vi "TrajectoryBegin.vi"(8 "error in (no error)":errorcluster) -> (0 "error out":errorcluster)   [LabVIEW 2023]
uses:
  TrajectoryGlobals.vi
  <vilib>/Rock Robotics/WPI/ThirdParty/JAS_Junk/TrajLib/Trajectory_Library.lvlib
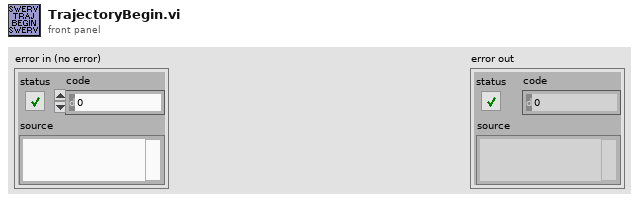
[diagram p1: front panel]
types:
  T1 = typedef "Trajectory_Library.lvlib/TRAJECTORY.ctl" = cluster{"TotalTImeSecs":dbl, "States":T2[]}
  T2 = typedef "Trajectory_Library.lvlib/TRAJ_STATE.ctl" = cluster{"TimeSeconds":dbl, "Velocity":dbl, "Acceleration":dbl, "POSE":T3, "Curvature":dbl}
  T3 = typedef "Trajectory_Library.lvlib/POSE2D.ctl" = cluster{"TRANSLATION":T4, "ROTATION":T5}
  T4 = typedef "Trajectory_Library.lvlib/TRANSLATION2D.ctl" = cluster{"X":dbl, "Y":dbl}
  T5 = typedef "Trajectory_Library.lvlib/ROTATION2D.ctl" = cluster{"VALUE":dbl, "COS":dbl, "SIN":dbl}
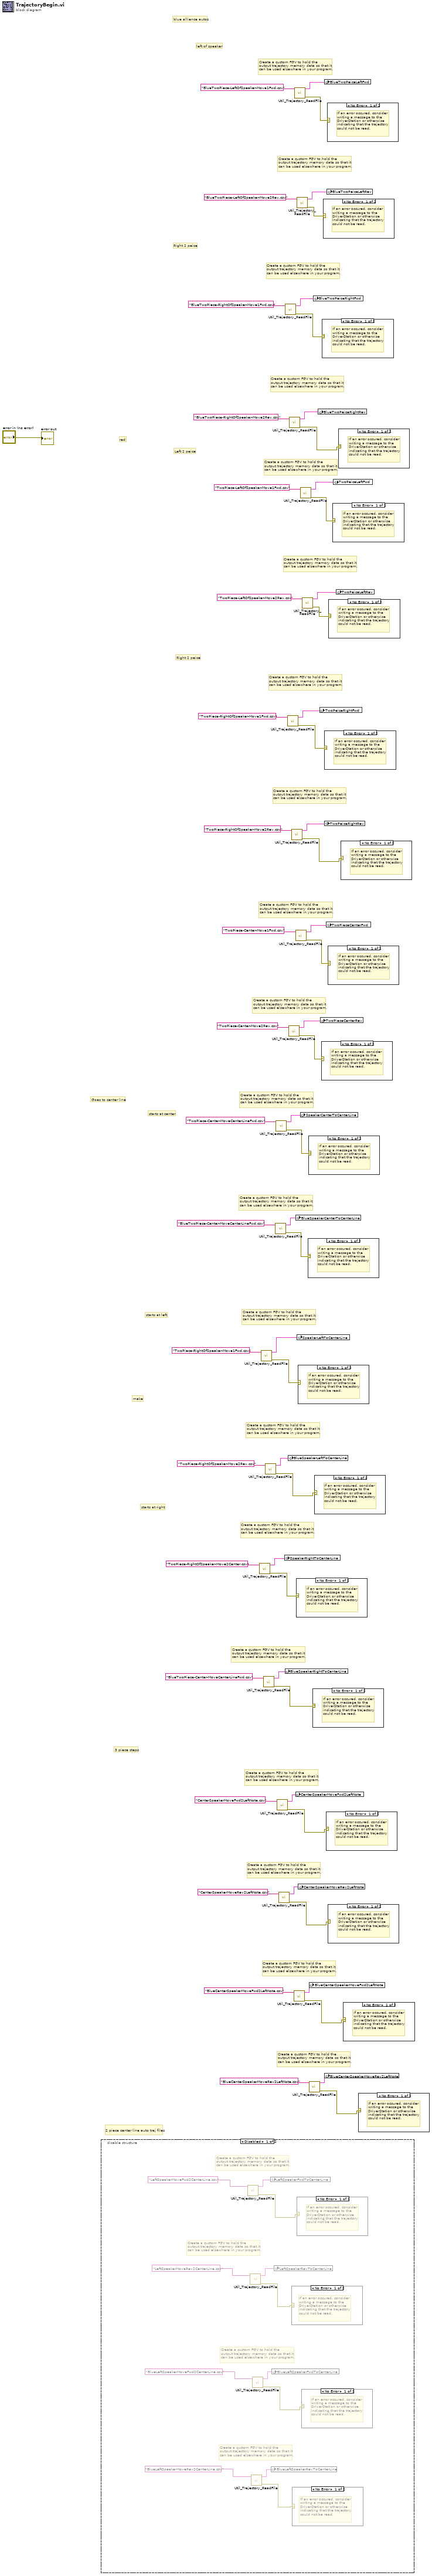
[diagram p0: block diagram]
diagram:
  # "2 piece center line auto traj files"
  # "Create a custom FGV to hold the \noutput trajectory memory data so that it\ncan be used elsewhere in your program."
  # "Create a custom FGV to hold the \noutput trajectory memory data so that it\ncan be used elsewhere in your program."
  # "Create a custom FGV to hold the \noutput trajectory memory data so that it\ncan be used elsewhere in your program."
  # "3 piece steps"
  # "Create a custom FGV to hold the \noutput trajectory memory data so that it\ncan be used elsewhere in your program."
  # "make"
  # "Create a custom FGV to hold the \noutput trajectory memory data so that it\ncan be used elsewhere in your program."
  # "Create a custom FGV to hold the \noutput trajectory memory data so that it\ncan be used elsewhere in your program."
  # "Create a custom FGV to hold the \noutput trajectory memory data so that it\ncan be used elsewhere in your program."
  # "Create a custom FGV to hold the \noutput trajectory memory data so that it\ncan be used elsewhere in your program."
  # "starts at right"
  # "starts at left"
  # "starts at center"
  # "Goes to center line"
  # "Create a custom FGV to hold the \noutput trajectory memory data so that it\ncan be used elsewhere in your program."
  # "Create a custom FGV to hold the \noutput trajectory memory data so that it\ncan be used elsewhere in your program."
  # "Create a custom FGV to hold the \noutput trajectory memory data so that it\ncan be used elsewhere in your program."
  # "Create a custom FGV to hold the \noutput trajectory memory data so that it\ncan be used elsewhere in your program."
  # "red"
  # "Right 2 peice"
  # "Create a custom FGV to hold the \noutput trajectory memory data so that it\ncan be used elsewhere in your program."
  # "Create a custom FGV to hold the \noutput trajectory memory data so that it\ncan be used elsewhere in your program."
  # "Create a custom FGV to hold the \noutput trajectory memory data so that it\ncan be used elsewhere in your program."
  # "Create a custom FGV to hold the \noutput trajectory memory data so that it\ncan be used elsewhere in your program."
  # "left of speaker"
  # "blue allience autos"
  # "Right 2 peice"
  # "Left 2 peice"
  # "Create a custom FGV to hold the \noutput trajectory memory data so that it\ncan be used elsewhere in your program."
  # "Create a custom FGV to hold the \noutput trajectory memory data so that it\ncan be used elsewhere in your program."
  # "Create a custom FGV to hold the \noutput trajectory memory data so that it\ncan be used elsewhere in your program."
  # "Create a custom FGV to hold the \noutput trajectory memory data so that it\ncan be used elsewhere in your program."
  n1 = disable-structure shown="Disabled" {
    frame Disabled {
      # "Create a custom FGV to hold the \noutput trajectory memory data so that it\ncan be used elsewhere in your program."
      # "Create a custom FGV to hold the \noutput trajectory memory data so that it\ncan be used elsewhere in your program."
      # "Create a custom FGV to hold the \noutput trajectory memory data so that it\ncan be used elsewhere in your program."
      # "Create a custom FGV to hold the \noutput trajectory memory data so that it\ncan be used elsewhere in your program."
      n2 = call <vilib>:"Util_Trajectory_ReadFile.vi"("FileName"="LeftSpeakerMoveFwd2CenterLine.csv") -> ("error out"=w71:errorcluster, "outTRAJECTORY"=w72:T1)  [unwired: 8 in, 1 out]
      n3 = call <vilib>:"Util_Trajectory_ReadFile.vi"("FileName"="LeftSpeakerMoveRev2CenterLine.csv") -> ("error out"=w68:errorcluster, "outTRAJECTORY"=w69:T1)  [unwired: 8 in, 1 out]
      n4 = call <vilib>:"Util_Trajectory_ReadFile.vi"("FileName"="BlueLeftSpeakerMoveRev2CenterLine.csv") -> ("error out"=w62:errorcluster, "outTRAJECTORY"=w63:T1)  [unwired: 8 in, 1 out]
      n5 = call <vilib>:"Util_Trajectory_ReadFile.vi"("FileName"="BlueLeftSpeakerMoveFwd2CenterLine.csv") -> ("error out"=w65:errorcluster, "outTRAJECTORY"=w66:T1)  [unwired: 8 in, 1 out]
      n6 = global write "TrajectoryGlobals.vi" "LeftSpeakerFwdToCenterLine"(w72) -> ()
      n7 = global write "TrajectoryGlobals.vi" "BlueLeftSpeakerRevToCenterLine"(w63) -> ()
      n8 = global write "TrajectoryGlobals.vi" "BlueLeftSpeakerFwdToCenterLine"(w66) -> ()
      n9 = global write "TrajectoryGlobals.vi" "LeftSpeakerRevToCenterLine"(w69) -> ()
      n10 = case shown="No Error" w68 {
        frame No Error {
          # "If an error occured, consider\nwriting a message to the\nDriverStation or otherwise\nindicating that the trajectory\ncould not be read."
        }
        frame Error {
        }
      }
      n11 = case shown="No Error" w62 {
        frame No Error {
          # "If an error occured, consider\nwriting a message to the\nDriverStation or otherwise\nindicating that the trajectory\ncould not be read."
        }
        frame Error {
        }
      }
      n12 = case shown="No Error" w71 {
        frame No Error {
          # "If an error occured, consider\nwriting a message to the\nDriverStation or otherwise\nindicating that the trajectory\ncould not be read."
        }
        frame Error {
        }
      }
      n13 = case shown="No Error" w65 {
        frame No Error {
          # "If an error occured, consider\nwriting a message to the\nDriverStation or otherwise\nindicating that the trajectory\ncould not be read."
        }
        frame Error {
        }
      }
    }
    frame Enabled {
    }
  }
  n14 = call <vilib>:"Util_Trajectory_ReadFile.vi"("FileName"="TwoPiece-RightOfSpeaker-Move2Center.csv") -> ("error out"=w22:errorcluster, "outTRAJECTORY"=w23:T1)  [unwired: 8 in, 1 out]
  n15 = call <vilib>:"Util_Trajectory_ReadFile.vi"("FileName"="TwoPiece-RightOfSpeaker-Move1Fwd.csv") -> ("error out"=w16:errorcluster, "outTRAJECTORY"=w17:T1)  [unwired: 8 in, 1 out]
  n16 = call <vilib>:"Util_Trajectory_ReadFile.vi"("FileName"="BlueTwoPiece-Center-MoveCenterLineFwd.csv") -> ("error out"=w19:errorcluster, "outTRAJECTORY"=w20:T1)  [unwired: 8 in, 1 out]
  n17 = call <vilib>:"Util_Trajectory_ReadFile.vi"("FileName"="TwoPiece-RightOfSpeaker-Move2Rev.csv") -> ("error out"=w13:errorcluster, "outTRAJECTORY"=w14:T1)  [unwired: 8 in, 1 out]
  n18 = call <vilib>:"Util_Trajectory_ReadFile.vi"("FileName"="BlueTwoPiece-Center-MoveCenterLineFwd.csv") -> ("error out"=w27:errorcluster, "outTRAJECTORY"=w25:T1)  [unwired: 8 in, 1 out]
  n19 = call <vilib>:"Util_Trajectory_ReadFile.vi"("FileName"="TwoPiece-Center-MoveCenterLineFwd.csv") -> ("error out"=w30:errorcluster, "outTRAJECTORY"=w28:T1)  [unwired: 8 in, 1 out]
  n20 = call <vilib>:"Util_Trajectory_ReadFile.vi"("FileName"="CenterSpeakerMoveFwd2LeftNote.csv") -> ("error out"=w10:errorcluster, "outTRAJECTORY"=w11:T1)  [unwired: 8 in, 1 out]
  n21 = call <vilib>:"Util_Trajectory_ReadFile.vi"("FileName"="CenterSpeakerMoveRev2LeftNote.csv") -> ("error out"=w7:errorcluster, "outTRAJECTORY"=w8:T1)  [unwired: 8 in, 1 out]
  n22 = global write "TrajectoryGlobals.vi" "SpeakerRightToCenterLine"(w23) -> ()
  n23 = global write "TrajectoryGlobals.vi" "BlueSpeakerRightToCenterLine"(w20) -> ()
  n24 = call <vilib>:"Util_Trajectory_ReadFile.vi"("FileName"="BlueTwoPiece-RightOfSpeaker-Move1Fwd.csv") -> ("error out"=w40:errorcluster, "outTRAJECTORY"=w41:T1)  [unwired: 8 in, 1 out]
  n25 = call <vilib>:"Util_Trajectory_ReadFile.vi"("FileName"="TwoPiece-RightOfSpeaker-Move1Fwd.csv") -> ("error out"=w52:errorcluster, "outTRAJECTORY"=w53:T1)  [unwired: 8 in, 1 out]
  n26 = global write "TrajectoryGlobals.vi" "BlueSpeakerLeftToCenterLine"(w14) -> ()
  n27 = call <vilib>:"Util_Trajectory_ReadFile.vi"("FileName"="TwoPiece-Center-Move2Rev.csv") -> ("error out"=w33:errorcluster, "outTRAJECTORY"=w31:T1)  [unwired: 8 in, 1 out]
  n28 = call <vilib>:"Util_Trajectory_ReadFile.vi"("FileName"="BlueTwoPiece-RightOfSpeaker-Move2Rev.csv") -> ("error out"=w37:errorcluster, "outTRAJECTORY"=w38:T1)  [unwired: 8 in, 1 out]
  n29 = call <vilib>:"Util_Trajectory_ReadFile.vi"("FileName"="TwoPiece-RightOfSpeaker-Move2Rev.csv") -> ("error out"=w49:errorcluster, "outTRAJECTORY"=w50:T1)  [unwired: 8 in, 1 out]
  n30 = call <vilib>:"Util_Trajectory_ReadFile.vi"("FileName"="BlueCenterSpeakerMoveFwd2LeftNote.csv") -> ("error out"=w4:errorcluster, "outTRAJECTORY"=w5:T1)  [unwired: 8 in, 1 out]
  n31 = call <vilib>:"Util_Trajectory_ReadFile.vi"("FileName"="BlueTwoPiece-LeftOfSpeaker-Move1Fwd.csv") -> ("error out"=w48:errorcluster, "outTRAJECTORY"=w46:T1)  [unwired: 8 in, 1 out]
  n32 = call <vilib>:"Util_Trajectory_ReadFile.vi"("FileName"="TwoPiece-Center-Move1Fwd.csv") -> ("error out"=w36:errorcluster, "outTRAJECTORY"=w34:T1)  [unwired: 8 in, 1 out]
  n33 = global write "TrajectoryGlobals.vi" "CenterSpeakerMoveFwd2LeftNote"(w11) -> ()
  n34 = global write "TrajectoryGlobals.vi" "BlueSpeakerCenterToCenterLine"(w25) -> ()
  n35 = case shown="No Error" w22 {
    frame No Error {
      # "If an error occured, consider\nwriting a message to the\nDriverStation or otherwise\nindicating that the trajectory\ncould not be read."
    }
    frame Error {
    }
  }
  n36 = call <vilib>:"Util_Trajectory_ReadFile.vi"("FileName"="BlueTwoPiece-LeftOfSpeaker-Move2Rev.csv") -> ("error out"=w43:errorcluster, "outTRAJECTORY"=w44:T1)  [unwired: 8 in, 1 out]
  n37 = global write "TrajectoryGlobals.vi" "SpeakerLeftToCenterLine"(w17) -> ()
  n38 = case shown="No Error" w16 {
    frame No Error {
      # "If an error occured, consider\nwriting a message to the\nDriverStation or otherwise\nindicating that the trajectory\ncould not be read."
    }
    frame Error {
    }
  }
  n39 = global write "TrajectoryGlobals.vi" "CenterSpeakerMoveRev2LeftNote"(w8) -> ()
  n40 = call <vilib>:"Util_Trajectory_ReadFile.vi"("FileName"="TwoPiece-LeftOfSpeaker-Move1Fwd.csv") -> ("error out"=w60:errorcluster, "outTRAJECTORY"=w58:T1)  [unwired: 8 in, 1 out]
  n41 = global write "TrajectoryGlobals.vi" "SpeakerCenterToCenterLine"(w28) -> ()
  n42 = call <vilib>:"Util_Trajectory_ReadFile.vi"("FileName"="TwoPiece-LeftOfSpeaker-Move2Rev.csv") -> ("error out"=w55:errorcluster, "outTRAJECTORY"=w56:T1)  [unwired: 8 in, 1 out]
  n43 = case shown="No Error" w27 {
    frame No Error {
      # "If an error occured, consider\nwriting a message to the\nDriverStation or otherwise\nindicating that the trajectory\ncould not be read."
    }
    frame Error {
    }
  }
  n44 = case shown="No Error" w30 {
    frame No Error {
      # "If an error occured, consider\nwriting a message to the\nDriverStation or otherwise\nindicating that the trajectory\ncould not be read."
    }
    frame Error {
    }
  }
  n45 = global write "TrajectoryGlobals.vi" "BlueCenterSpeakerMoveFwd2LeftNote"(w5) -> ()
  n46 = call <vilib>:"Util_Trajectory_ReadFile.vi"("FileName"="BlueCenterSpeakerMoveRev2LeftNote.csv") -> ("error out"=w1:errorcluster, "outTRAJECTORY"=w2:T1)  [unwired: 8 in, 1 out]
  n47 = case shown="No Error" w19 {
    frame No Error {
      # "If an error occured, consider\nwriting a message to the\nDriverStation or otherwise\nindicating that the trajectory\ncould not be read."
    }
    frame Error {
    }
  }
  n48 = global write "TrajectoryGlobals.vi" "BlueTwoPeiceRightFwd"(w41) -> ()
  n49 = case shown="No Error" w13 {
    frame No Error {
      # "If an error occured, consider\nwriting a message to the\nDriverStation or otherwise\nindicating that the trajectory\ncould not be read."
    }
    frame Error {
    }
  }
  n50 = global write "TrajectoryGlobals.vi" "BlueTwoPeiceRightRev"(w38) -> ()
  n51 = global write "TrajectoryGlobals.vi" "TwoPeiceRightFwd"(w53) -> ()
  n52 = global write "TrajectoryGlobals.vi" "TwoPieceCenterRev"(w31) -> ()
  n53 = case shown="No Error" w33 {
    frame No Error {
      # "If an error occured, consider\nwriting a message to the\nDriverStation or otherwise\nindicating that the trajectory\ncould not be read."
    }
    frame Error {
    }
  }
  n54 = case shown="No Error" w40 {
    frame No Error {
      # "If an error occured, consider\nwriting a message to the\nDriverStation or otherwise\nindicating that the trajectory\ncould not be read."
    }
    frame Error {
    }
  }
  n55 = case shown="No Error" w43 {
    frame No Error {
      # "If an error occured, consider\nwriting a message to the\nDriverStation or otherwise\nindicating that the trajectory\ncould not be read."
    }
    frame Error {
    }
  }
  n56 = global write "TrajectoryGlobals.vi" "BlueTwoPeiceLeftFwd"(w46) -> ()
  n57 = global write "TrajectoryGlobals.vi" "TwoPeiceRightRev"(w50) -> ()
  n58 = case shown="No Error" w52 {
    frame No Error {
      # "If an error occured, consider\nwriting a message to the\nDriverStation or otherwise\nindicating that the trajectory\ncould not be read."
    }
    frame Error {
    }
  }
  n59 = global write "TrajectoryGlobals.vi" "BlueCenterSpeakerMoveRev2LeftNote"(w2) -> ()
  n60 = case shown="No Error" w10 {
    frame No Error {
      # "If an error occured, consider\nwriting a message to the\nDriverStation or otherwise\nindicating that the trajectory\ncould not be read."
    }
    frame Error {
    }
  }
  n61 = global write "TrajectoryGlobals.vi" "TwoPieceCenterFwd"(w34) -> ()
  n62 = global write "TrajectoryGlobals.vi" "BlueTwoPeiceLeftRev"(w44) -> ()
  n63 = case shown="No Error" w48 {
    frame No Error {
      # "If an error occured, consider\nwriting a message to the\nDriverStation or otherwise\nindicating that the trajectory\ncould not be read."
    }
    frame Error {
    }
  }
  n64 = case shown="No Error" w36 {
    frame No Error {
      # "If an error occured, consider\nwriting a message to the\nDriverStation or otherwise\nindicating that the trajectory\ncould not be read."
    }
    frame Error {
    }
  }
  n65 = case shown="No Error" w7 {
    frame No Error {
      # "If an error occured, consider\nwriting a message to the\nDriverStation or otherwise\nindicating that the trajectory\ncould not be read."
    }
    frame Error {
    }
  }
  n66 = case shown="No Error" w55 {
    frame No Error {
      # "If an error occured, consider\nwriting a message to the\nDriverStation or otherwise\nindicating that the trajectory\ncould not be read."
    }
    frame Error {
    }
  }
  n67 = case shown="No Error" w60 {
    frame No Error {
      # "If an error occured, consider\nwriting a message to the\nDriverStation or otherwise\nindicating that the trajectory\ncould not be read."
    }
    frame Error {
    }
  }
  n68 = global write "TrajectoryGlobals.vi" "TwoPeiceLeftFwd"(w58) -> ()
  n69 = global write "TrajectoryGlobals.vi" "TwoPeiceLeftRev"(w56) -> ()
  n70 = case shown="No Error" w37 {
    frame No Error {
      # "If an error occured, consider\nwriting a message to the\nDriverStation or otherwise\nindicating that the trajectory\ncould not be read."
    }
    frame Error {
    }
  }
  n71 = case shown="No Error" w49 {
    frame No Error {
      # "If an error occured, consider\nwriting a message to the\nDriverStation or otherwise\nindicating that the trajectory\ncould not be read."
    }
    frame Error {
    }
  }
  n72 = case shown="No Error" w4 {
    frame No Error {
      # "If an error occured, consider\nwriting a message to the\nDriverStation or otherwise\nindicating that the trajectory\ncould not be read."
    }
    frame Error {
    }
  }
  n73 = case shown="No Error" w1 {
    frame No Error {
      # "If an error occured, consider\nwriting a message to the\nDriverStation or otherwise\nindicating that the trajectory\ncould not be read."
    }
    frame Error {
    }
  }
  "error out" <- "error in (no error)"
